vi "TCP Listen.vi"(6 "resolve remote address (T)":bool=TRUE, 7 "net address":u32, 8 "error in (no error)":errorcluster, 9 "timeout ms (wait forever: -1)":i32=-1, 10 "port":u16, 11 "service name":string) -> (0 "error out":errorcluster, 1 "remote port":u16, 2 "remote address":string, 3 "connection ID":refnum<k5>, 5 "listener ID":refnum<k5>)   [LabVIEW 2020]
doc: "Creates a listener and waits for an accepted TCP network connection at the specified <B>port</B>."
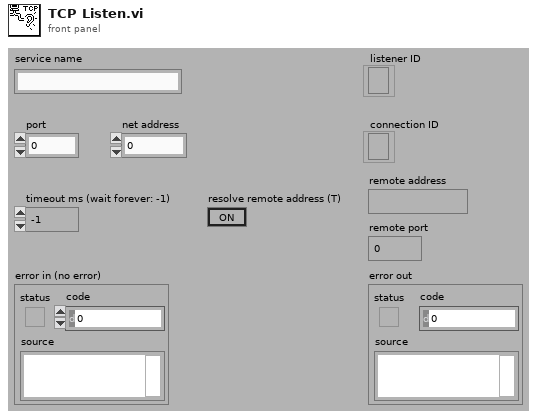
[diagram p1: front panel]
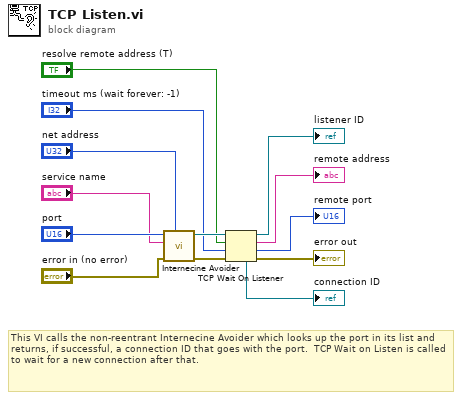
[diagram p0: block diagram]
diagram:
  # "This VI calls the non-reentrant Internecine Avoider which looks up the port in its list and returns, if successful, a connection ID that goes with the port.  TCP Wait on Listen is called to wait for a new connection after that."
  n1 = call <vilib>:"Internecine Avoider.vi"("net address"="net address", "error in"="error in (no error)", "service name"="service name", "port"="port") -> ("error out"=w9:errorcluster, "connection ID"=w10:refnum<k5>)  [unwired: 6 out]
  n2 = TCP Wait On Listener(8:w9, 9:"timeout ms (wait forever: -1)", 10:"resolve remote address (T)", 11:w10) -> (0:→"error out":errorcluster, 1:→"remote port":u16, 2:→"remote address":string, 3:→"listener ID":refnum<k5>, 4:→"connection ID":refnum<k5>)
